vi "prog.vi"() -> ()   [LabVIEW 2017]
uses:
  <vilib>/Utility/error.llb/DialogType.ctl
  Instance          13 12Saved   prog .vi
  Instance          11 12Saved   prog .vi
  Instance          12 12Saved   prog .vi
  DAQmx Create Channel (AO-Voltage-Basic).vi
  DAQmx Create Channel (AI-Voltage-Basic).vi
  DAQmx Write (Analog DBL 1Chan 1Samp).vi
  DAQmx Read (Analog 1D DBL NChan 1Samp).vi
  <vilib>/Utility/file.llb/Write To Spreadsheet File (DBL).vi
panel:
  in  "Case Constant\n(See Context Help) 2":bool=TRUE
  in  "Case Constant\n(See Context Help)":bool=TRUE
  in  "RadB factor":dbl
  out "RadB - gain 2":dbl
  out "RadA - gain 3":dbl=-1.9275641423518846
  in  "ms to wait":u32=6
  in  "LASERS ON":bool
  in  "CO2 limits":cluster{dbl, dbl}(slide)={2.04, 4.0} caption="CO2\nmax" scale=0.0..5.0 scale format="%#_2g"
  in  "CO2 DC":tag="Dev1/ao1" caption="CO2 power ao1"
  out "PID out":dbl=1.0 format="%.2f"
  in  "file path":path=path "c:/ilan/log.txt"
  in  "Sound tol.":dbl=444.0
  out "XY Graph":cluster{"Y":dbl[], "Y":dbl[]}[](graph)
  in  "START":bool
  in  "Display skip":i16=10
  out "Temperature":dbl=26.87605238540693 format="%#_4g"
  out "b":dbl=38.68797484161706 caption="Const - b" format="%#.2g"
  out "a":dbl=6.127901114511302 caption="Slope - a" format="%#.2g"
  in  "set point":dbl=60.0 format="%.2f"
  in  "D":dbl(slide)=0.0989795918367347 scale=0.0..0.1 scale format="%#_3g"
  in  "I":dbl(slide)=1.040816326530612 scale=0.0..2.0 scale format="%#_3g"
  in  "P":dbl(slide)=0.4897959183673469 scale=0.0..2.0 scale format="%#_3g"
  in  "Rad. channel":tag="Dev1/ai3" caption="rad channel ai0"
  out "f samp.":dbl=162.51438180369945 format="%#.2g"
  in  "stop":bool
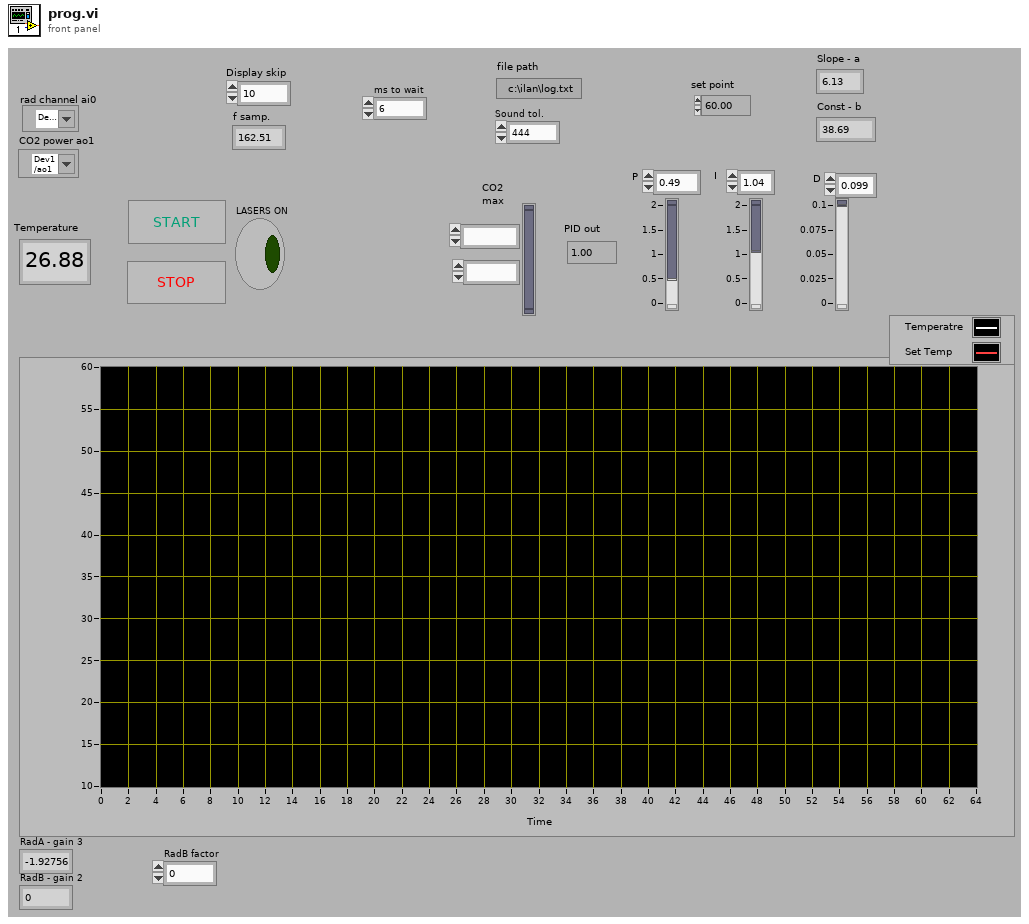
[diagram p1: front panel]
types:
  T1 = typedef "DialogType.ctl" = u16
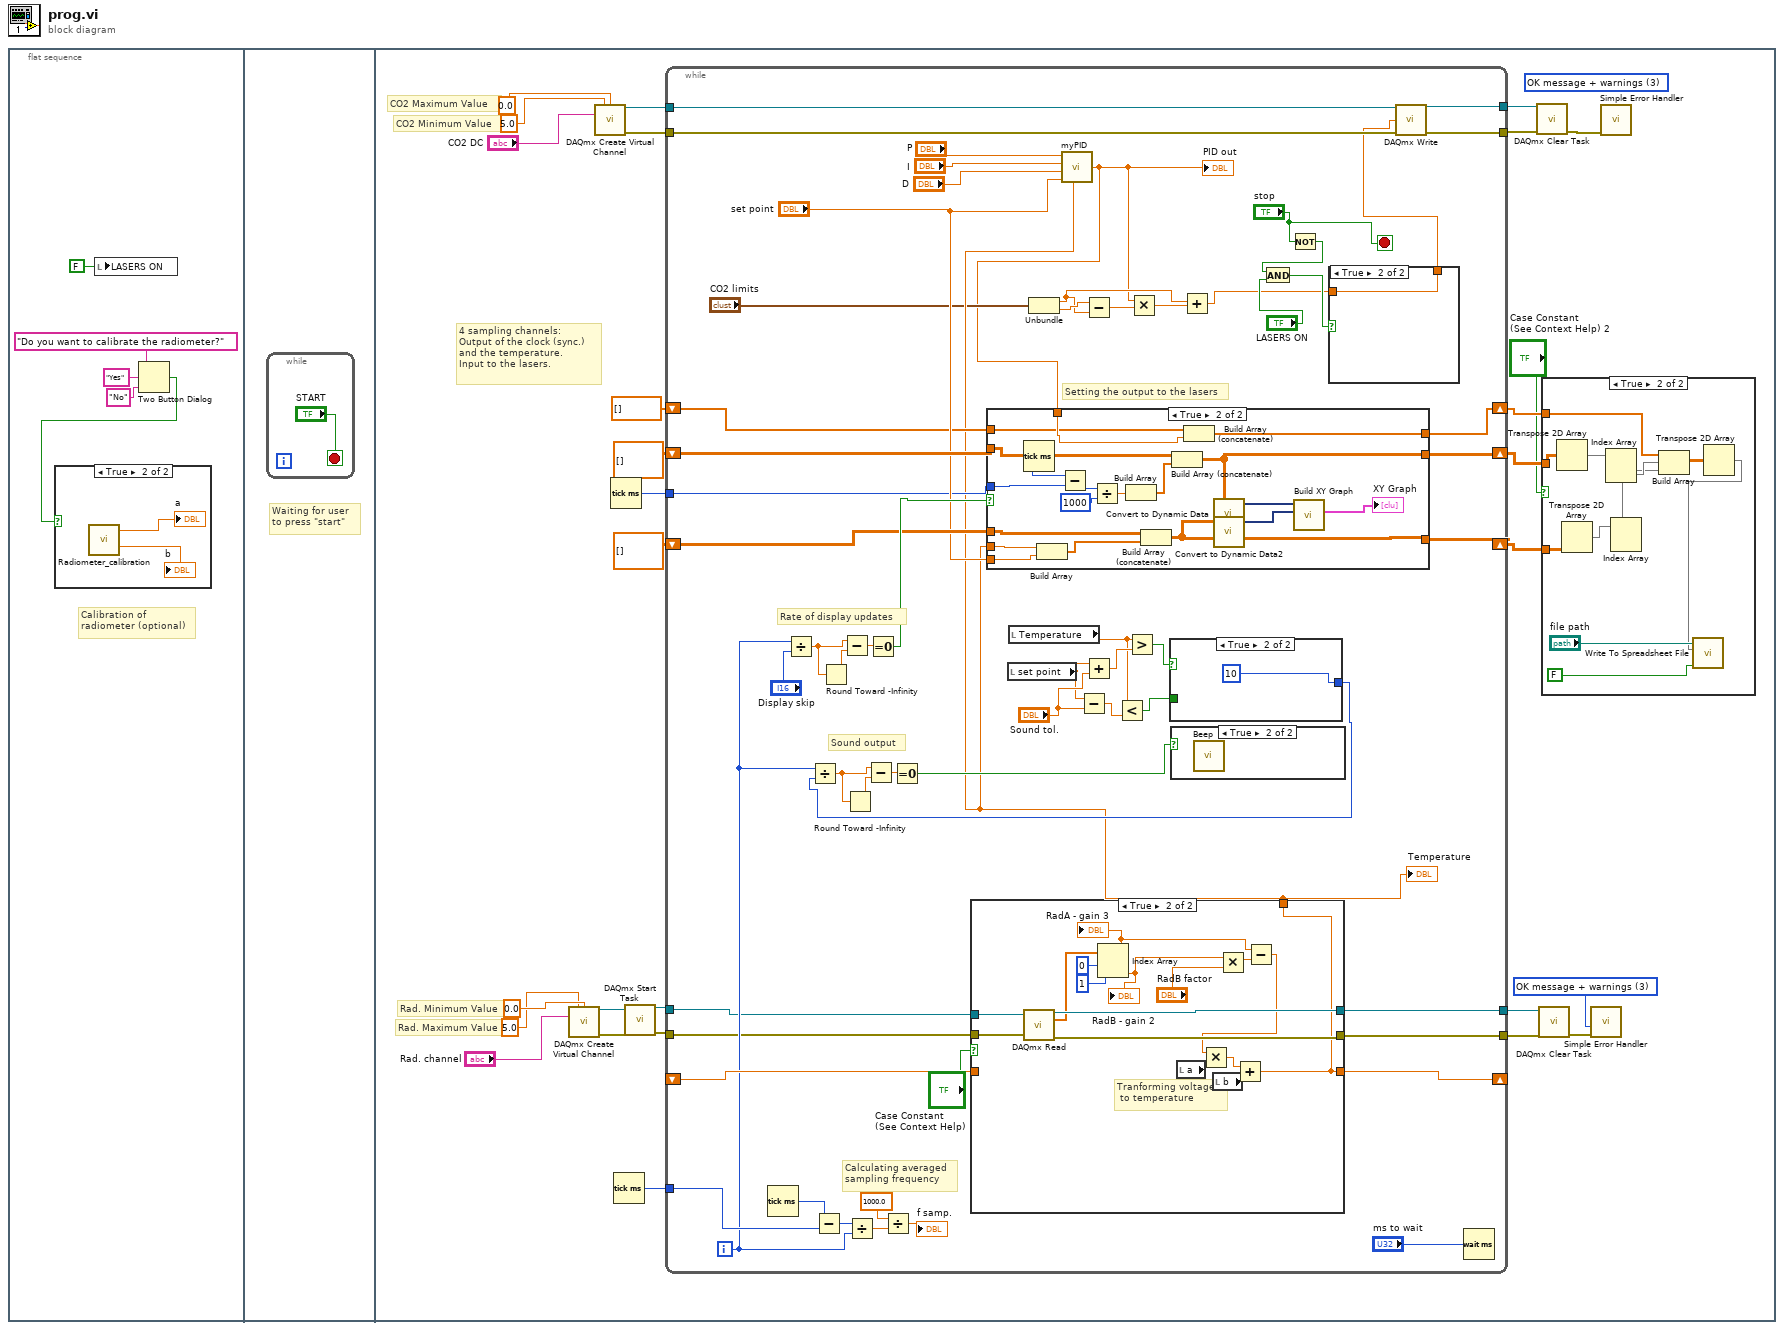
[diagram p0: block diagram]
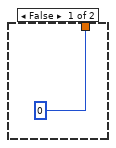
[diagram p4: hidden frame]
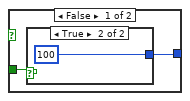
[diagram p5: hidden frame]
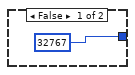
[diagram p6: hidden frame]
diagram:
  n1 = flat-sequence {
    frame #0 {
      # "Calibration of \nradiometer (optional)"
      n2 = local write "LASERS ON"(FALSE ("LASERS ON")) -> ()
      n3 = Two Button Dialog(message="Do you want to calibrate the radiometer?", 1:"No" ("F button name (\"Cancel\")"), 2:"Yes" ("T button name (\"OK\")")) -> (T button?=w2:bool)
      n4 = case shown="True" w2 {
        frame False {
        }
        frame True {
          n5 = call "Radiometer_calibration.vi"() -> ("b=T_2+a*V_2"=→"b":dbl, "a=(T_2-T_1)/(V_2-V_1)"=→"a":dbl)  [unwired: 4 in]
        }
      }
    }
    frame #1 {
      # "Waiting for user \nto press \"start\""
      n6 = while {
        stop <- "START" stop-if-true
      }
    }
    frame #2 {
      (unwired) T1 3 items=["no dialog", "OK message", "continue or stop message", "OK message + warnings", "continue/stop + warnings"] ("type of dialog (OK msg:1)")
      w32 = T1 3 items=["no dialog", "OK message", "continue or stop message", "OK message + warnings", "continue/stop + warnings"] ("type of dialog (OK msg:1)")
      # "CO2 Maximum Value"
      # "CO2 Minimum Value"
      # "4 sampling channels:\nOutput of the clock (sync.)\nand the temperature.\nInput to the lasers."
      # "Rad. Maximum Value"
      # "Rad. Minimum Value"
      n7 = call-poly "DAQmx Create Virtual Channel.vi"("maximum value"=5.0 ("Rad. Maximum Value"), "minimum value"=0.0 ("Rad. Minimum Value"), "physical channels"="Rad. channel") -> ("task out"=w13:refnum<k21>, "error out"=w12:errorcluster)  [unwired: 11 in]
      n8 = call-poly "DAQmx Create Virtual Channel.vi"("maximum value"=5.0 ("GaAsMaximum Value"), "minimum value"=0.0 ("GaAs Minimum Value"), "physical channels"="CO2 DC") -> ("task out"=w20:refnum<k21>, "error out"=w19:errorcluster)  [unwired: 11 in]
      n9 = Tick Count (ms)() -> (millisecond timer value=w28:u32)
      n10 = Tick Count (ms)() -> (millisecond timer value=w29:u32)
      n11 = call "DAQmx Start Task.vi"("task/channels in"=w13, "error in"=w12) -> ("task out"=w11:refnum<k21>, "error out"=w10:errorcluster)  [unwired: 12 in]
      n12 = while {
        tunnel: [w106] -> w31
        tunnel: [w105] -> w30
        tunnel: w29 -> [w104]
        shift-right: [w97] -> _
        shift-left: _ -> [w96]
        shift-right: [w88] -> w15
        shift-left: dbl[][] [] -> [w89]
        shift-right: [w87] -> w25
        shift-left: dbl[][] [] -> [w86]
        tunnel: w28 -> [w56]
        tunnel: w20 -> [w72]
        tunnel: w19 -> [w71]
        tunnel: [w70] -> w18
        tunnel: [w69] -> w17
        shift-right: [w66] -> w14
        shift-left: dbl[] [] -> [w67]
        tunnel: w11 -> [w58]
        tunnel: w10 -> [w57]
        i -> [w81]
        stop <- "stop" stop-if-true
        # "Sound output"
        # "Calculating averaged\nsampling frequency"
        # "Rate of display updates"
        # "Setting the output to the lasers"
        n13 = Tick Count (ms)() -> (millisecond timer value=w101:u32)
        n14 = Divide(x=w81, y="Display skip") -> (x/y=w93:dbl)
        n15 = Subtract(x=w101, y=w104) -> (x-y=w90:u32)
        n16 = Round Toward -Infinity(1:w93) -> (0:w92:dbl)
        n17 = Subtract(x=w93, y=w92) -> (x-y=w94:dbl)
        n18 = Divide(x=w90, y=w81) -> (x/y=w107:dbl)
        n19 = Equal To 0?(x=w94) -> (x = 0?=w91:bool)
        n20 = Divide(x=1000.0, y=w107) -> (x/y=→"f samp.":dbl)
        n21 = case shown="True" "Case Constant\n(See Context Help)" {
          tunnel: [w138 w155] -> w106
          tunnel: [w137 w154] -> w105
          tunnel: [w139 w140] -> w55
          tunnel: [w139 w140] -> w97
          tunnel: w96 -> [w139 _]
          tunnel: w58 -> [w138 w150]
          tunnel: w57 -> [w137 w149]
          frame False {
          }
          frame True {
            # "Tranforming voltage\n to temperature"
            n22 = call-poly "DAQmx Read.vi"("task/channels in"=w150, "error in"=w149) -> ("task out"=w155:refnum<k21>, "data"=w146:dbl[], "error out"=w154:errorcluster)  [unwired: 11 in]
            n23 = Index Array(array=w146, index #1=0 ("index"), index #2=1 ("index")) -> (element #1=w145:dbl, element #2=w142:dbl)
            "RadA - gain 3" <- w145
            "RadB - gain 2" <- w142
            n24 = local read "a"() -> (w151:dbl)
            n25 = local read "b"() -> (w152:dbl)
            n26 = Multiply(x=w142, y="RadB factor") -> (x*y=w143:dbl)
            n27 = Subtract(x=w145, y=w143) -> (x-y=w144:dbl)
            n28 = Multiply(x=w144, y=w151) -> (x*y=w153:dbl)
            n29 = Add(x=w153, y=w152) -> (x+y=w140:dbl)
          }
        }
        "Temperature" <- w55
        n30 = local read "set point"() -> (w79:dbl)
        n31 = local read "Temperature"() -> (w75:dbl)
        n32 = Unbundle("CO2 limits") -> (w51:dbl, w53:dbl)
        n33 = call "myPID.vi"("P"="P", "I"="I", "D"="D", "set point"="set point", "process variable"=w55) -> ("output value"=w49:dbl)
        "PID out" <- w49
        n34 = case shown="True" w91 {
          tunnel: w55 -> [_ w122]
          tunnel: w56 -> [_ w135]
          tunnel: w89 -> [w117 w134]
          tunnel: [w117 w124] -> w88
          tunnel: "set point" -> [_ w121]
          tunnel: [w116 w128] -> w87
          tunnel: w86 -> [w116 w131]
          tunnel: w49 -> [_ w120]
          tunnel: w67 -> [w115 w119]
          tunnel: [w115 w118] -> w66
          frame False {
          }
          frame True {
            n35 = Tick Count (ms)() -> (millisecond timer value=w136:u32)
            n36 = Build Array(w122, w121) -> (w129:dbl[])
            n37 = Subtract(x=w136, y=w135) -> (x-y=w133:u32)
            n38 = Divide(x=w133, y=u32 1000) -> (x/y=w126:dbl)
            n39 = Build Array(w126, w126) -> (w125:dbl[])
            n40 = Build Array (concatenate)(w131, w129) -> (w128:dbl[][])
            n41 = Build Array (concatenate)(w134, w125) -> (w124:dbl[][])
            n42 = Build Array (concatenate)(w119, w120) -> (w118:dbl[])
            n43 = call "Convert to Dynamic Data"("2D Array"=w124) -> ("Dynamic Data Type"=w123:dynamicdata)  [unwired: 3 in]
            n44 = call "Convert to Dynamic Data2"("2D Array"=w128) -> ("Dynamic Data Type"=w127:dynamicdata)  [unwired: 3 in]
            n45 = call "Build XY Graph"("Y Input"=w127, "X Input"=w123) -> ("XY Graph"=→"XY Graph":cluster{"Y":dbl[], "Y":dbl[]}[])  [unwired: 8 in, 1 out]
          }
        }
        n46 = Subtract(x=w79, y="Sound tol.") -> (x-y=w78:dbl)
        n47 = Subtract(x=w53, y=w51) -> (x-y=w54:dbl)
        n48 = Add(x=w79, y="Sound tol.") -> (x+y=w76:dbl)
        n49 = Less?(x=w75, y=w78) -> (x < y?=w74:bool)
        n50 = Greater?(x=w75, y=w76) -> (0:w77:bool)
        n51 = Multiply(x=w49, y=w54) -> (x*y=w52:dbl)
        n52 = case shown="True" w77 {
          tunnel: w74 -> [w111 _]
          tunnel: [w110 i16 10 ("sound const")] -> w59
          frame False {
            n53 = case shown="True" w111 {
              tunnel: [i16 32767 ("sound const") i16 100 ("sound const")] -> w110
              frame False {
              }
              frame True {
              }
            }
          }
          frame True {
          }
        }
        n54 = Divide(x=w81, y=w59) -> (x/y=w83:dbl)
        n55 = Round Toward -Infinity(1:w83) -> (0:w82:dbl)
        n56 = Subtract(x=w83, y=w82) -> (x-y=w84:dbl)
        n57 = Equal To 0?(x=w84) -> (x = 0?=w68:bool)
        n58 = case shown="True" w68 {
          frame False {
          }
          frame True {
            n59 = call <vilib>:"Beep.vi"() -> ()  [unwired: 12 in]
          }
        }
        n60 = Add(x=w51, y=w52) -> (x+y=w48:dbl)
        n61 = Not(x="stop") -> (.not. x?=w61:bool)
        n62 = And(x=w61, y="LASERS ON") -> (x .and. y?=w62:bool)
        n63 = case shown="True" w62 {
          tunnel: w48 -> [_ w109]
          tunnel: [0 w109] -> w64
          frame False {
          }
          frame True {
          }
        }
        n64 = call-poly "DAQmx Write.vi"("task/channels in"=w72, "data"=w64, "error in"=w71) -> ("task out"=w69:refnum<k21>, "error out"=w70:errorcluster)  [unwired: 10 in, 1 out]
        n65 = Wait (ms)(milliseconds to wait="ms to wait") -> ()  [unwired: 1 out]
      }
      n66 = call "DAQmx Clear Task.vi"("task in"=w17, "error in"=w18) -> ("error out"=w24:errorcluster)  [unwired: 13 in]
      n67 = call "DAQmx Clear Task.vi"("task in"=w31, "error in"=w30) -> ("error out"=w33:errorcluster)  [unwired: 13 in]
      n68 = case shown="True" "Case Constant\n(See Context Help) 2" {
        tunnel: w25 -> [_ w45]
        tunnel: w15 -> [_ w39]
        tunnel: w14 -> [_ w37]
        frame False {
        }
        frame True {
          n69 = Transpose 2D Array(2D array=w39) -> (transposed array=w38:dbl[][])
          n70 = Transpose 2D Array(2D array=w45) -> (transposed array=w44:dbl[][])
          n71 = Index Array(array=w38) -> (element=w43:dbl[])  [unwired: 2 in]
          n72 = Index Array(array=w44) -> (element=w42:dbl[])  [unwired: 2 in]
          n73 = Build Array(w37, w43, w42) -> (w41:dbl[][])
          n74 = Transpose 2D Array(2D array=w41) -> (transposed array=w40:dbl[][])
          n75 = call-poly <vilib>:"Write To Spreadsheet File.vi"("append to file? (new file:F)"=FALSE, "2D data"=w40, "file path (dialog if empty)"="file path") -> ()  [unwired: 5 in, 1 out]
        }
      }
      n76 = call <vilib>:"Simple Error Handler.vi"("type of dialog (OK msg:1)"=w32, "error in (no error)"=w33) -> ()  [unwired: 3 in, 5 out]
      n77 = call <vilib>:"Simple Error Handler.vi"("error in (no error)"=w24) -> ()  [unwired: 4 in, 5 out]
    }
  }
